vi "DemoReadAnalog.vi"() -> ()   [LabVIEW 2009]
uses:
  <vilib>/NXT/Block Support/NXT_InputPort.ctl
  <vilib>/NXT/Dual Mode Library/Waits/Wait_Num(msec).vi
  <vilib>/NXT/Dual Mode Library/Display/drawText.vi
panel:
  in  "stop":bool
  # "HiTechnic Experimenter's Kit\n\nDemo Read Analog\n\n(c) HiTechnic 2011"
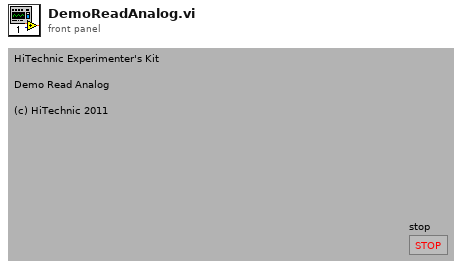
[diagram p1: front panel]
types:
  T1 = typedef "NXT_InputPort.ctl" = u8
  T2 = typedef "LVHSConnector.ctl" = cluster{"error":errorcluster, "address":string, "NXT #":i32, "Show Error":bool, "Connection":u16}
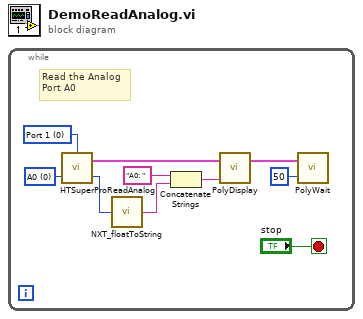
[diagram p0: block diagram]
diagram:
  n1 = while {
    stop <- "stop" stop-if-true
    w1 = T1 0 items=["Port 1", "Port 2", "Port 3", "Port 4"] ("Port")
    w9 = u8 0 items=["A0", "A1", "A2", "A3"] ("Analog Port")
    # "Read the Analog\nPort A0"
    n2 = call "HTSuperProReadAnalog.vi"("Analog Port"=w9, "Port"=w1) -> ("Analog Value"=w4:i16, "NXT"=w8:T2)  [unwired: 2 in]
    n3 = call <vilib>:"NXT_floatToString.vi"("number"=w4) -> ("string"=w5:string)
    n4 = Concatenate Strings("A0: " ("string"), w5) -> (w7:string)
    n5 = call-poly <vilib>:"PolyDisplay.vi"("Text"=w7, "NXT"=w8) -> ("NXT"=w2:T2)  [unwired: 2 in]
    n6 = call-poly <vilib>:"PolyWait.vi"("Time (100 msec)"=u32 50, "NXT"=w2) -> ()  [unwired: 2 in, 1 out]
  }
